vi "UDP-ImgReceiver.vi"() -> ()   [LabVIEW 2020]
doc: "The UDP protocol differs from TCP in that there is no error-checking with the packets of information that are sent, and thus no guarantee whatsoever that an intended recipient will actually receive a given piece of data.\n\nUDP does offer the ability to \"broadcast\" data across a network--simply specify an IP Address of all ones (255.255.255.255) to attempt to broadcast information network-wide. Keep in mind that routers and other network hardware will generally refuse to forward the broadcast beyond certain points, so the extent of the broadcast will in practice be limited."
uses:
  <vilib>/vision/Image Controls.llb/IMAQ Image.ctl
panel:
  out "Image":T1(plugin-control)
  in  "Stop":bool
  # "UDP - Image Receiver"
  # "Instruction:\n1. Run UDP Sender;\n2. Run Image Receiver.\n3. see the images transfered\n to image reveiver."
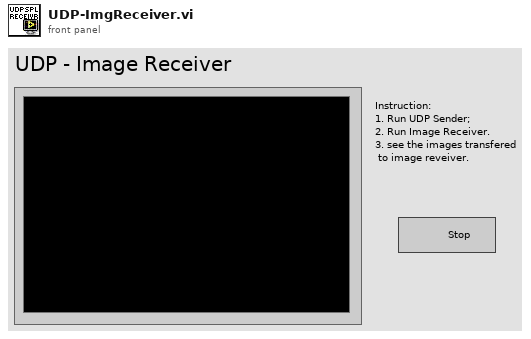
[diagram p1: front panel]
types:
  T1 = typedef "IMAQ Image.ctl" = refnum<image>
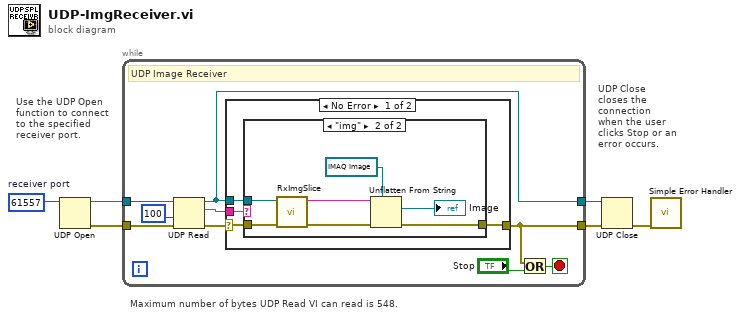
[diagram p0: block diagram]
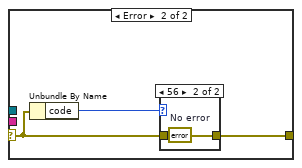
[diagram p3: hidden frame]
diagram:
  w1 = u16 61557  # receiver port
  # "UDP Close closes the connection when the user clicks Stop or an error occurs."
  # "Use the UDP Open function to connect to the specified receiver port."
  # "Maximum number of bytes UDP Read VI can read is 548."
  n1 = UDP Open(11:w1) -> (port=w2:refnum<k16>, 0:w3:errorcluster)  [unwired: 4 in, 1 out]
  n2 = while {
    tunnel: w2 -> [w15]
    tunnel: [w7] -> w6
    tunnel: w3 -> [w12]
    tunnel: [w8] -> w4
    stop <- w13 stop-if-true
    # "UDP Image Receiver"
    n3 = UDP Read(connection ID=w15, timeout ms (25000)=100, 8:w12) -> (data out=w10:string, error out=w9:errorcluster, 3:w7:refnum<k16>)  [unwired: 3 out]
    n4 = case shown="No Error" w9 {
      selector: w9 -> [w19 w29]
      tunnel: w10 -> [w17 _]
      tunnel: [w18 w28] -> w8
      tunnel: w7 -> [w16 _]
      frame No Error {
        # "Sender sent data. Update the image"
        n5 = case shown="\"img\"" w17 {
          tunnel: w19 -> [w20 w27]
          tunnel: [w20 w22] -> w18
          tunnel: w16 -> [_ w26]
          frame Default {
          }
          frame "img" {
            n6 = call "RxImgSlice.vi"("error in"=w27, "Conn"=w26) -> ("error out"=w23:errorcluster, "Data"=w21:string)  [unwired: 8 in]
            n7 = Unflatten From String(type=T1 refnum ("Image"), binary string=w21, error in (no error)=w23) -> (value=→"Image":T1, error out=w22:errorcluster)  [unwired: 2 in, 1 out]
          }
        }
      }
      frame Error {
        # "Sender did not send data. Ignore timeout error and keep waiting."
        n8 = Unbundle By Name(w29) -> ("code"=w30:i32)
        n9 = case shown="56" w30 {
          tunnel: w29 -> [w31 _]
          tunnel: [w31 w32] -> w28
          frame Default {
          }
          frame 56 {
            w32 = errorcluster {"status"=FALSE, "code"=0, "source"=""}  # No error
          }
        }
      }
    }
    n10 = Or(x=w8, y="Stop") -> (x .or. y?=w13:bool)
  }
  n11 = UDP Close(connection ID=w6, 8:w4) -> (error out=w5:errorcluster)  [unwired: 1 out]
  n12 = call <vilib>:"Simple Error Handler.vi"("error in (no error)"=w5) -> ()  [unwired: 1 in, 8 out]
